vi "test Variant Run-Time Error.vi"(8 "error in (no error)":errorcluster, 11 "TestCase in":refnum<class "Malleable Tests.lvclass">) -> (0 "error out":errorcluster, 3 "TestCase out":refnum<class "Malleable Tests.lvclass">)   [LabVIEW 2020, in "Memory Manager Tests.lvlib" / "Malleable Tests.lvclass"]
uses:
  Malleable Tests.lvclass
  <vilib>/addons/_JKI Toolkits/VI Tester/TestCase.llb/TestCase.lvclass
  Malleable Type Tests/Malleable Type Tests.lvclass
  C:/Program Files (x86)/National Instruments/LabVIEW 2020/vi.lib/addons/_JKI Toolkits/VI Tester/TestCase.llb/TestCase.lvclass
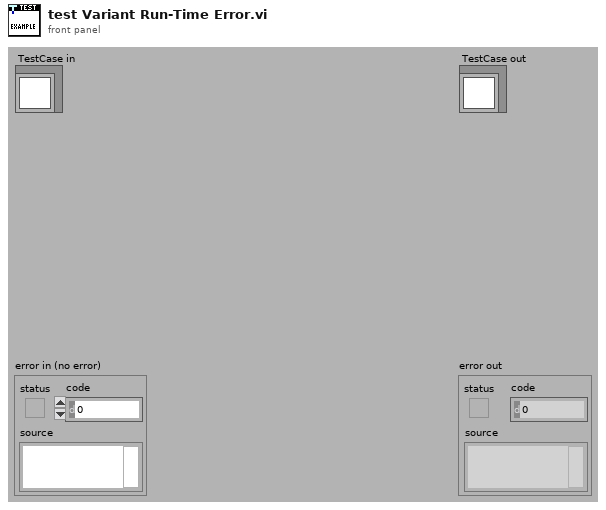
[diagram p1: front panel]
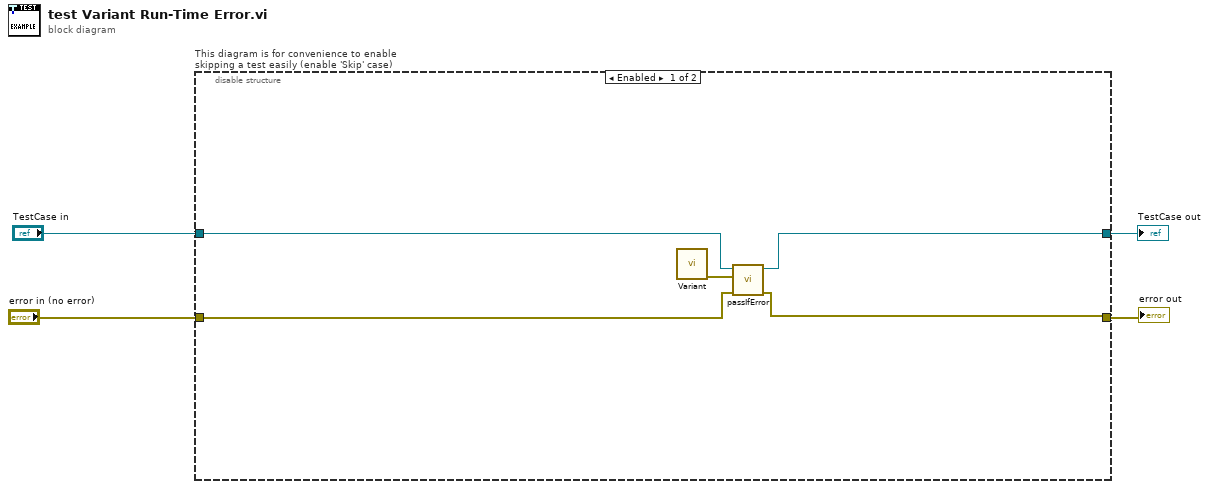
[diagram p0: block diagram]
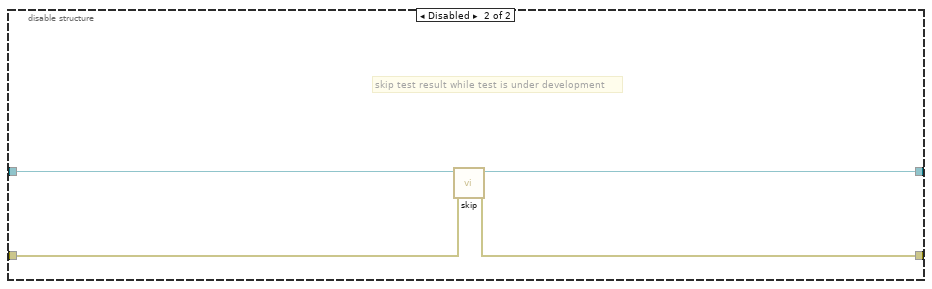
[diagram p2: hidden frame]
diagram:
  n1 = disable-structure "This diagram is for convenience to enable skipping a test easily (enable 'Skip' case)" shown="Enabled" {
    disable-tunnel: "TestCase in" -> [w9 w13]
    disable-tunnel: [w8 w11] -> w1
    disable-tunnel: [w7 w12] -> w3
    disable-tunnel: "error in (no error)" -> [w6 w10]
    frame Enabled {
      n2 = call "Variant.vi"() -> ("error out"=w5:errorcluster)  [unwired: 11 in]
      n3 = call-dynamic "passIfError.vi"("error in (no error)"=w6, "error"=w5, "TestCase in"=w9) -> ("error out"=w7:errorcluster, "TestCase out"=w8:refnum<class "Malleable Tests.lvclass">)  [unwired: 7 in]
    }
    frame Disabled {
      # "skip test result while test is under development"
      n4 = call <vilib>:"skip.vi"("error in (no error)"=w10, "TestCase in"=w13) -> ("error out"=w12:errorcluster, "TestCase out"=w11:refnum<class "Malleable Tests.lvclass">)  [unwired: 8 in]
    }
  }
  "error out" <- w3
  "TestCase out" <- w1
